vi "ImageComposer.vi"(2 "Y":i32, 4 "HEIGHT":i32, 5 "X":i32, 6 "WIDTH":i32, 7 "BACK_IMAGE":path, 9 "SAVE":bool, 10 "FORE_IMAGE":path, 11 "PICTURE IN":refnum<vi>) -> (0 "ERROR OUT":errorcluster, 3 "PICTURE OUT":picture)   [LabVIEW 2015]
uses:
  System.Drawing
  <vilib>/picture/picture.llb/Draw True-Color Pixmap.vi
  <vilib>/wsapi/NI_WebServices.lvlib
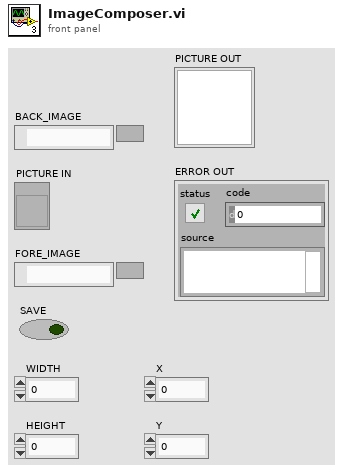
[diagram p1: front panel]
types:
  T1 = typedef "imagedata.ctl" = cluster{"image type":i32, "image depth":i32, "image":u8[], "mask":u8[], "colors":u32[], "Rectangle":cluster{"left":i16, "top":i16, "right":i16, "bottom":i16}}
  T2 = cluster{"left":i16, "top":i16, "right":i16, "bottom":i16}
  T3 = typedef "LVBoundsTypeDef.ctl" = cluster{"Width":u32, "Height":u32}
  T4 = enum16{"open", "replace", "create", "open or create", "replace or create", "replace or create with confirmation"}
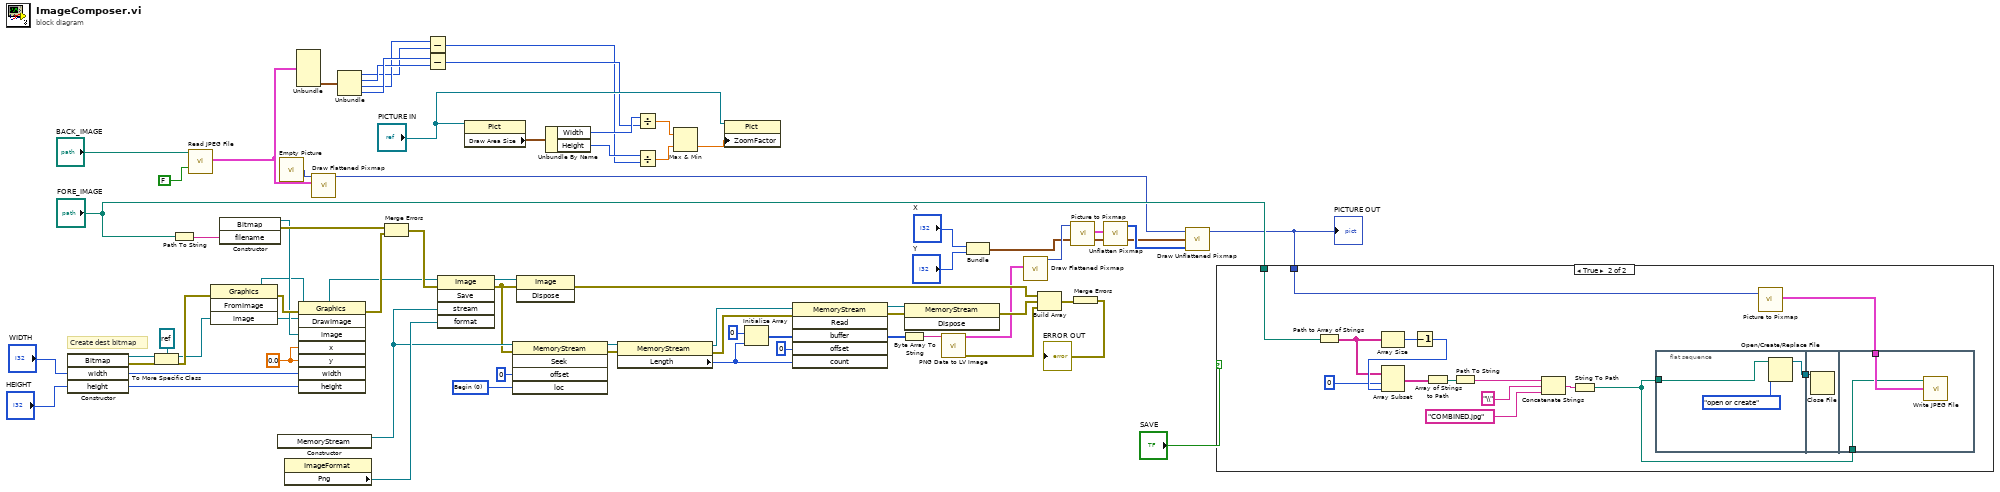
[diagram p0: block diagram]
diagram:
  w27 = 0 items=["Begin", "Current", "End"] ("loc")
  w19 = sgl 0.0 ("x")
  # "Create dest bitmap"
  n1 = constructor class="Bitmap"("width"="WIDTH", "height"="HEIGHT") -> (reference out=w21:refnum<k24>, error out=w45:errorcluster)  [unwired: 3 in, 3 out]
  n2 = To More Specific Class(target class=refnum<k24> refnum, reference=w21, error in=w45) -> (specific class reference=w39:refnum<k24>, error out=w46:errorcluster)
  n3 = Path To String(path="FORE_IMAGE") -> (string=w52:string)
  n4 = call <vilib>:"Read JPEG File.vi"("use 8 bit color table"=FALSE, "path to JPEG file"="BACK_IMAGE") -> ("image data"=w8:T1)  [unwired: 7 in, 2 out]
  n5 = invoke class="Graphics" method="FromImage"(error in=w46, "image"=w39) -> (error out=w47:errorcluster, "FromImage"=w22:refnum<k24>)  [unwired: 2 in, 2 out]
  n6 = constructor class="Bitmap"("filename"=w52) -> (reference out=w44:refnum<k24>, error out=w48:errorcluster)  [unwired: 3 in, 2 out]
  n7 = constructor class="MemoryStream"() -> (reference out=w51:refnum<k24>)  [unwired: 3 in, 2 out]
  n8 = call "Empty Picture"() -> ("empty picture"=w18:picture)
  n9 = property class="ImageFormat"() -> ("Png"=w53:refnum<k24>)  [unwired: 2 in, 2 out]
  n10 = Unbundle(w8) -> ("Rectangle"=w7:T2)  [unwired: 5 out]
  n11 = invoke class="Graphics" method="DrawImage"(reference=w22, error in=w47, "image"=w44, "x"=w19, "y"=w19, "width"="WIDTH", "height"="HEIGHT") -> (error out=w49:errorcluster)  [unwired: 1 in, 7 out]
  n12 = call <vilib>:"Draw Flattened Pixmap.vi"("image data"=w8, "picture"=w18) -> ("new picture"=w17:picture)  [unwired: 7 in]
  n13 = Unbundle(w7) -> ("left"=w1:i16, "top"=w5:i16, "right"=w2:i16, "bottom"=w6:i16)
  n14 = Merge Errors(w48, w49) -> (w50:errorcluster)
  n15 = Subtract(x=w2, y=w1) -> (x-y=w3:i16)
  n16 = Subtract(x=w6, y=w5) -> (x-y=w4:i16)
  n17 = invoke class="Image" method="Save"(reference=w39, error in=w50, "stream"=w51, "format"=w53) -> (reference out=w23:refnum<k24>, error out=w36:errorcluster)  [unwired: 1 in, 3 out]
  n18 = property on="Property Node" class="Pict"(reference="PICTURE IN") -> ("Draw Area Size"=w55:T3)  [unwired: 1 in, 2 out]
  n19 = invoke class="MemoryStream" method="Seek"(reference=w51, error in=w36, "offset"=i64 0, "loc"=w27) -> (reference out=w24:refnum<k24>, error out=w25:errorcluster)  [unwired: 1 in, 3 out]
  n20 = invoke class="Image" method="Dispose"(reference=w23, error in=w36) -> (error out=w42:errorcluster)  [unwired: 1 in, 2 out]
  n21 = Unbundle By Name(w55) -> ("Width"=w56:u32, "Height"=w57:u32)
  n22 = property class="MemoryStream"(reference=w24, error in=w25) -> (reference out=w29:refnum<k24>, error out=w30:errorcluster, "Length"=w32:i64)
  n23 = Divide(x=w56, y=w4) -> (x/y=w58:dbl)
  n24 = Divide(x=w57, y=w3) -> (x/y=w59:dbl)
  n25 = Max & Min(x=w58, y=w59) -> (min(x,y)=w60:dbl)  [unwired: 1 out]
  n26 = property on="Property Node" class="Pict"(reference="PICTURE IN", "ZoomFactor"=w60) -> ()  [unwired: 1 in, 2 out]
  n27 = Initialize Array(u8 0 ("element"), w32) -> (w31:u8[])
  n28 = invoke class="MemoryStream" method="Read"(reference=w29, error in=w30, "buffer"=w31, "offset"=0, "count"=w32) -> (reference out=w34:refnum<k24>, error out=w35:errorcluster, "buffer"=w37:u8[])  [unwired: 1 in, 3 out]
  n29 = Byte Array To String(unsigned byte array=w37) -> (string=w40:string)
  n30 = invoke class="MemoryStream" method="Dispose"(reference=w34, error in=w35) -> (error out=w38:errorcluster)  [unwired: 1 in, 2 out]
  n31 = call <vilib>:"PNG Data to LV Image.vi"("png data"=w40) -> ("error out"=w41:errorcluster, "image data"=w13:T1)  [unwired: 9 in]
  n32 = Bundle("X"="X", "Y"="Y") -> (w10:cluster{"X":i32, "Y":i32})  [unwired: 1 in]
  n33 = call <vilib>:"Draw Flattened Pixmap.vi"("image data"=w13) -> ("new picture"=w54:picture)  [unwired: 8 in]
  n34 = Build Array(w42, w38, w41) -> (w43:errorcluster[])
  n35 = call <vilib>:"Picture to Pixmap.vi"("picture"=w54) -> ("image data"=w14:T1)  [unwired: 9 in, 1 out]
  n36 = Merge Errors(w43) -> (→"ERROR OUT":errorcluster)
  n37 = call <vilib>:"Unflatten Pixmap.vi"("image data"=w14) -> ("24-bit pixmap"=w15:u32[][])  [unwired: 4 in, 6 out]
  n38 = call-poly <vilib>:"Draw Unflattened Pixmap.vi"("picture"=w17, "top left point(0, 0)"=w10, "data (RGB format)"=w15) -> ("new picture"=w9:picture)  [unwired: 6 in]
  "PICTURE OUT" <- w9
  n39 = case shown="True" "SAVE" {
    tunnel: "FORE_IMAGE" -> [_ w74]
    tunnel: w9 -> [_ w69]
    frame False {
    }
    frame True {
      n40 = Path to Array of Strings(0:w74) -> (2:w80:string[])  [unwired: 1 out]
      n41 = Array Size(array=w80) -> (size(s)=w76:i32)
      n42 = Decrement(x=w76) -> (x-1=w81:i32)
      n43 = Array Subset(array=w80, index=0, length=w81) -> (w77:string[])
      n44 = Array of Strings to Path(0:w77) -> (2:w78:path)  [unwired: 1 in]
      n45 = Path To String(path=w78) -> (string=w79:string)
      n46 = Concatenate Strings(w79, "\\" ("string"), "COMBINED.jpg" ("string")) -> (w82:string)
      n47 = String To Path(string=w82) -> (path=w71:path)
      n48 = flat-sequence {
        tunnel: w71 -> [w85]
        tunnel: [w83] -> w70
        tunnel: w70 -> [w86]
        tunnel: w71 -> [w87]
        tunnel: w68 -> [w88]
        frame #0 {
          n49 = Open/Create/Replace File(file path (use dialog)=w85, operation (0:open)=T4."open or create") -> (refnum out=w83:refnum<file>)  [unwired: 4 in, 2 out]
        }
        frame #1 {
          n50 = Close File(refnum=w86) -> ()  [unwired: 1 in, 2 out]
        }
        frame #2 {
          n51 = call <vilib>:"Write JPEG File.vi"("image data"=w88, "path to JPEG file"=w87) -> ()  [unwired: 8 in, 2 out]
        }
      }
      n52 = call <vilib>:"Picture to Pixmap.vi"("picture"=w69) -> ("image data"=w68:T1)  [unwired: 9 in, 1 out]
    }
  }
